vi "M-686 Send Command.vi"(0 "VISA Ref":refnum<visa-resource-name>, 2 "Wait for Reply (T)":bool=TRUE, 7 "Command":string, 11 "Error In":errorcluster) -> (4 "VISA Ref Dup":refnum<visa-resource-name>, 8 "Reply":string, 13 "Cmd Success":bool, 15 "Error Out":errorcluster)   [LabVIEW 2020]
uses:
  <vilib>/Utility/error.llb/whitespace.ctl
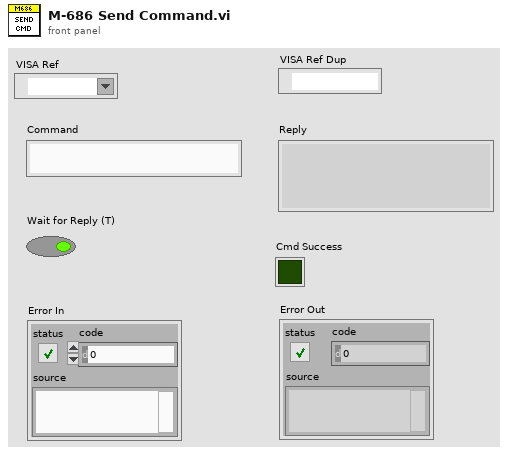
[diagram p1: front panel]
types:
  T1 = typedef "whitespace.ctl" = u16
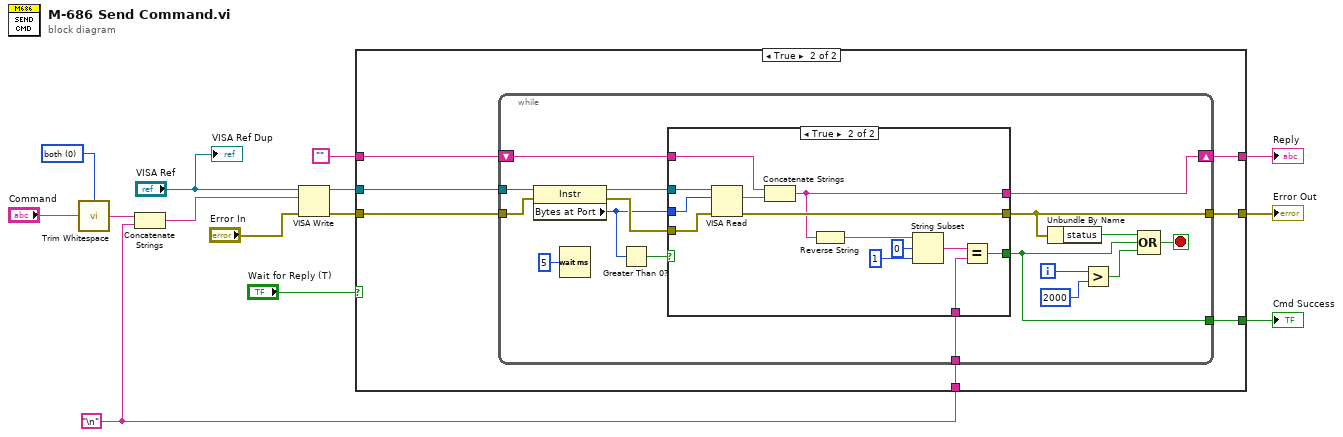
[diagram p0: block diagram]
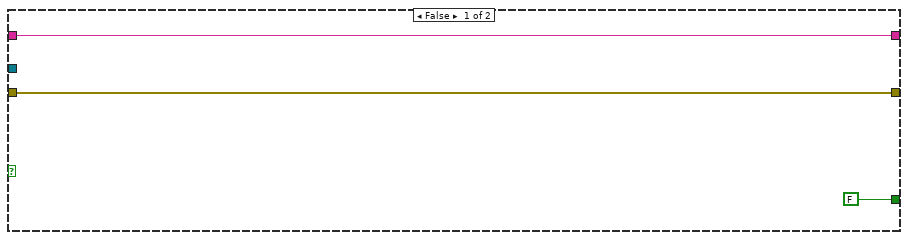
[diagram p2: hidden frame]
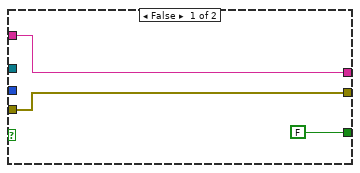
[diagram p3: hidden frame]
diagram:
  w3 = "\n"
  w13 = T1 0 items=["both", "start of string", "end of string"] ("location (both)")
  n1 = call <vilib>:"Trim Whitespace.vi"("string"="Command", "location (both)"=w13) -> ("trimmed string"=w12:string)
  n2 = Concatenate Strings(w12, w3) -> (w11:string)
  n3 = VISA Write(VISA resource name="VISA Ref", write buffer=w11, error in (no error)="Error In") -> (VISA resource name out=w10:refnum<visa-resource-name>, error out=w9:errorcluster)  [unwired: 1 out]
  n4 = case shown="True" "Wait for Reply (T)" {
    tunnel: w10 -> [_ w20]
    tunnel: w9 -> [w17 w19]
    tunnel: "" -> [w16 w24]
    tunnel: [w16 w23] -> w2
    tunnel: [w17 w22] -> w5
    tunnel: w3 -> [_ w21]
    tunnel: [FALSE w18] -> w1
    frame False {
    }
    frame True {
      n5 = while {
        tunnel: w20 -> [w41]
        tunnel: w19 -> [w40]
        shift-right: [w29] -> w23
        shift-left: w24 -> [w30]
        tunnel: [w27] -> w22
        tunnel: w21 -> [w26]
        tunnel: [w25] -> w18
        i -> [w39]
        stop <- w36 stop-if-true
        n6 = property class="Instr"(reference=w41, error in=w40) -> (reference out=w32:refnum<visa-resource-name>, error out=w33:errorcluster, "Bytes at Port"=w31:u32)
        n7 = Wait (ms)(milliseconds to wait=u32 5) -> ()  [unwired: 1 out]
        n8 = Greater Than 0?(x=w31) -> (x > 0?=w34:bool)
        n9 = case shown="True" w34 {
          tunnel: w33 -> [w44 w56]
          tunnel: w32 -> [_ w57]
          tunnel: w31 -> [_ w55]
          tunnel: w30 -> [w42 w54]
          tunnel: [w42 w51] -> w29
          tunnel: [w44 w52] -> w27
          tunnel: [FALSE w47] -> w25
          tunnel: w26 -> [_ w46]
          frame False {
          }
          frame True {
            n10 = VISA Read(VISA resource name=w57, byte count=w55, error in (no error)=w56) -> (read buffer=w53:string, error out=w52:errorcluster)  [unwired: 2 out]
            n11 = Concatenate Strings(w54, w53) -> (w51:string)
            n12 = Reverse String(1:w51) -> (0:w45:string)
            n13 = String Subset(string=w45, offset (0)=0, length (rest)=1 ("length (rest)")) -> (substring=w48:string)
            n14 = Equal?(x=w48, y=w46) -> (x = y?=w47:bool)
          }
        }
        n15 = Unbundle By Name(w27) -> ("status"=w28:bool)
        n16 = Greater?(x=w39, y=2000) -> (0:w37:bool)
        n17 = Compound Arithmetic op=OR(w28, w25, w37) -> (w36:bool)
      }
    }
  }
  "Reply" <- w2
  "Error Out" <- w5
  "Cmd Success" <- w1
  "VISA Ref Dup" <- "VISA Ref"
